vi "get channels.vi"(11 "Missing Plugin configuration in":refnum<class "Missing Plugin configuration.lvclass">) -> (2 "channels":refnum<class "TBM channel.lvclass">[](array[class]), 3 "Missing Plugin configuration out":refnum<class "Missing Plugin configuration.lvclass">)   [LabVIEW 2014, in "PL Framework Configuration Tool.lvlib" / "Missing Plugin configuration.lvclass"]
doc: "Returns an array of all Channels currently added to this configuration object."
uses:
  Missing Plugin configuration.lvclass
  <vilib>/NI/Tag Bus Module Framework/channel/TBM channel.lvclass
  Missing Plugin configuration.lvclass/Missing Plugin configuration.ctl
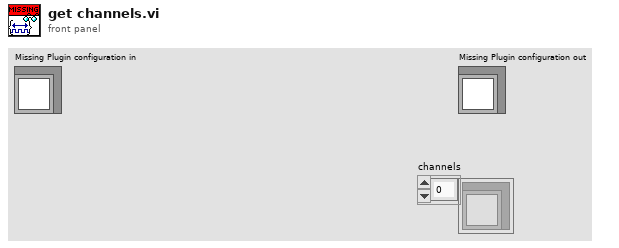
[diagram p1: front panel]
types:
  T1 = typedef "PL Framework Configuration Tool.lvlib/Missing Plugin configuration.lvclass/Line.ctl" = cluster{"channel":refnum<class "TBM channel.lvclass">}
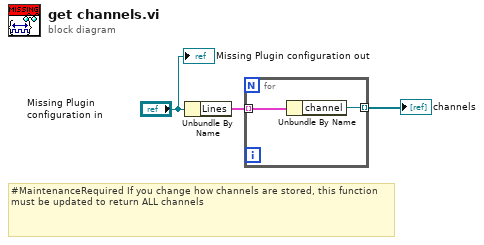
[diagram p0: block diagram]
diagram:
  # "#MaintenanceRequired If you change how channels are stored, this function must be updated to return ALL channels"
  n1 = Unbundle By Name("Missing Plugin configuration in") -> ("Lines"=w2:T1[])
  n2 = for {
    tunnel: w2 -> [w5] mode=indexing
    tunnel: [w4] -> w1 mode=indexing
    n3 = Unbundle By Name(w5) -> ("channel"=w4:refnum<class "TBM channel.lvclass">)
  }
  "channels" <- w1
  "Missing Plugin configuration out" <- "Missing Plugin configuration in"
